vi "Main.vi"() -> ()   [LabVIEW 2020, in "Main_Process.lvlib"]
uses:
  Main_Process.lvlib
  Controls/Edit Button.ctl
  Controls/Stop Button.ctl
  Controls/Start Button.ctl
  Controls/Main Loop Data.ctl
  Task_Management/Task_Management.lvclass
  Internal Message Library/Internal Messaging Library.lvlib
panel:
  in  "Stop Button":T1
  in  "Start Button":T2
  in  "Button":T3
  in  "Add Button":bool
  in  "Projects":i32(listbox)
  in  "Tasks":i32(listbox)
  in  "TimeCard Listbox":i32(listbox)
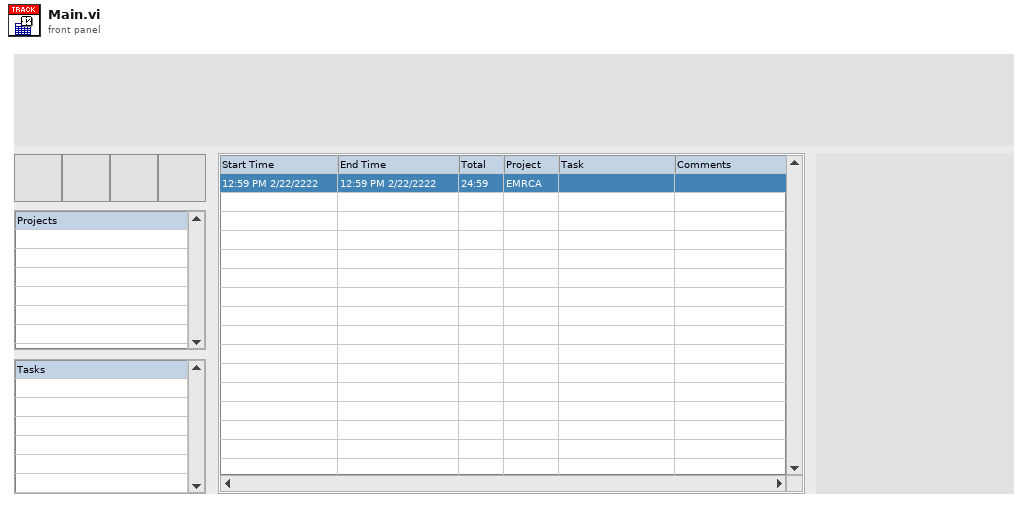
[diagram p1: front panel]
types:
  T1 = typedef "Stop Button.ctl" = bool
  T2 = typedef "Start Button.ctl" = bool
  T3 = typedef "Edit Button.ctl" = bool
  T4 = typedef "Main_Process.lvlib/Main Loop Data.ctl" = cluster{"Task_Management.lvclass":refnum<class "Task_Management.lvclass">}
  T5 = typedef "Main_Process.lvlib/Internal Messaging Library.lvlib/Message.ctl" = enum16{"Initialize", "Exit", "Error", "Load Data", "Add Time Entry", "Modify Time Entry", "Delete Time Entry"}
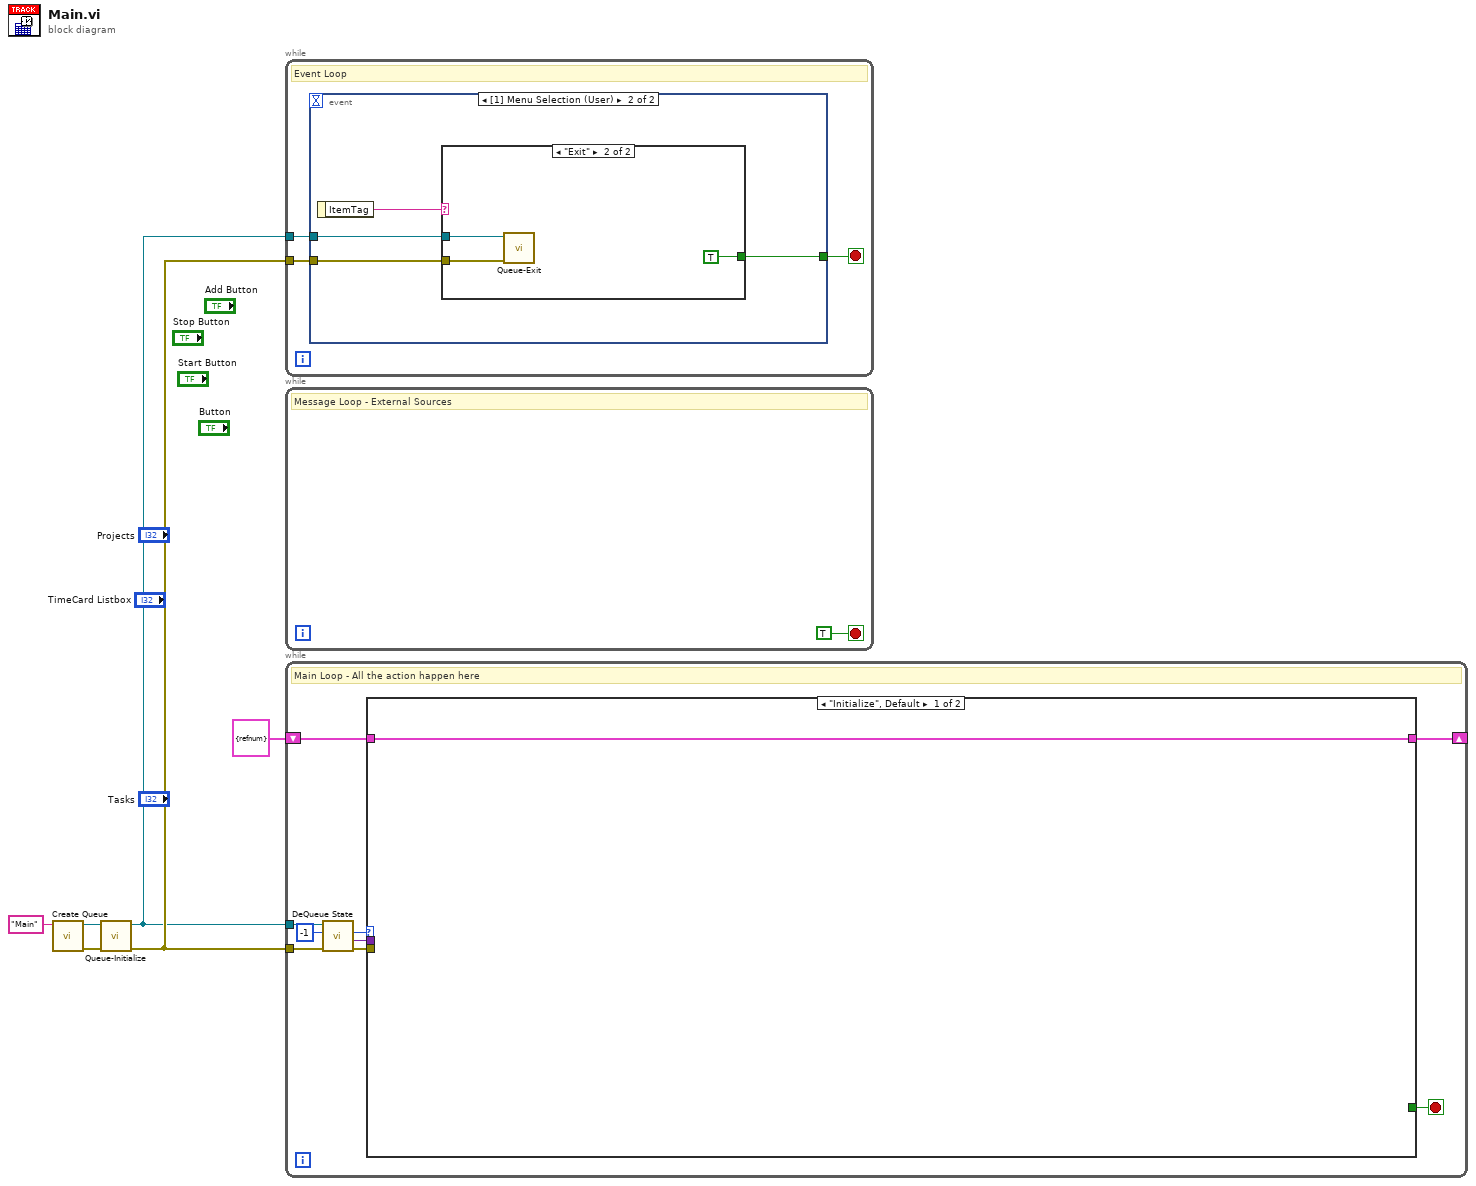
[diagram p0: block diagram]
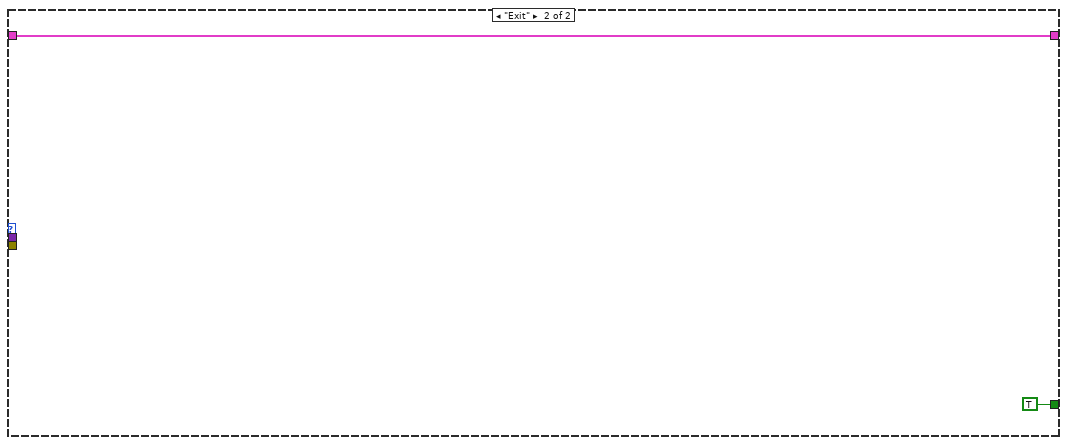
[diagram p2: hidden frame]
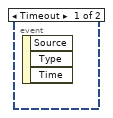
[diagram p3: hidden frame]
diagram:
  n1 = call "Create Queue.vi"("Process Name"="Main") -> ("error out"=w3:errorcluster, "queue out"=w4:refnum<queue>)  [unwired: 9 in]
  n2 = call "Queue-Initialize.vi"("error in"=w3, "Queue In"=w4) -> ("error out"=w2:errorcluster, "Queue Out"=w1:refnum<queue>)  [unwired: 8 in]
  n3 = while {
    tunnel: w2 -> [w8]
    tunnel: w1 -> [w7]
    stop <- w9 stop-if-true
    # "Event Loop"
    n4 = event shown="[1] Menu Selection (User)" {
      selector: _ -> [_ _]
      dyn-events: _ -> [_ _]
      timeout: _ -> [_ _]
      tunnel: [_ w12] -> w9
      tunnel: w8 -> [_ w11]
      tunnel: w7 -> [_ w10]
      event Timeout {
        n5 = event-data() -> ()  [unwired: 1 in, 3 out]
      }
      event Menu Selection (User) {
        n6 = event-data() -> ("ItemTag"=w13:string)  [unwired: 1 in]
        n7 = case shown="\"Exit\"" w13 {
          tunnel: [_ TRUE] -> w12
          tunnel: w11 -> [_ w15]
          tunnel: w10 -> [_ w14]
          frame Default {
          }
          frame "Exit" {
            n8 = call "Queue-Exit.vi"("error in"=w15, "Queue In"=w14) -> ()  [unwired: 8 in, 2 out]
          }
        }
      }
    }
  }
  n9 = while {
    stop <- TRUE stop-if-true
    # "Message Loop - External Sources"
  }
  n10 = while {
    shift-right: [w24] -> _
    shift-left: T4 {"Task_Management.lvclass"=refnum} ("Main Loop Data") -> [w25]
    tunnel: w1 -> [w23]
    tunnel: w2 -> [w22]
    stop <- w26 stop-if-true
    # "Main Loop - All the action happen here"
    n11 = call "DeQueue State.vi"("error in"=w22, "Timeout (-1)"=-1, "queue in"=w23) -> ("error out"=w18:errorcluster, "Message Data"=w19:variant, "Message"=w20:T5)  [unwired: 5 in, 1 out]
    n12 = case shown="\"Initialize\", Default" w20 {
      tunnel: [_ TRUE] -> w26
      tunnel: w25 -> [w27 w28]
      tunnel: [w27 w28] -> w24
      tunnel: w19 -> [_ _]
      tunnel: w18 -> [_ _]
      frame "Initialize", Default {
      }
      frame "Exit" {
      }
    }
  }
